vi "mqttClient_ModelController.vi"() -> ()   [LabVIEW 2019]
uses:
  DUT/state -- cluster.ctl
  <vilib>/LabVIEW Open Source Project/OpenSerializer JKI JSON/Serializer.JSON.lvclass
  C:/Program Files (x86)/National Instruments/LabVIEW 2019/vi.lib/LabVIEW Open Source Project/OpenSerializer/Serializer/Serializer.lvclass
  DUT/target -- cluster.ctl
  <vilib>/LabVIEW Open Source Project/MQTT Connection/MQTT_Base/Base Class/MQTT_Base.lvclass/MQTT_Base.ctl
  <vilib>/LabVIEW Open Source Project/MQTT Client/Client class/Client.lvclass/Client.ctl
  <vilib>/LabVIEW Open Source Project/MQTT Control Packets/Control Packets/ControlPacket/QualityOfService -- enum.ctl
  <vilib>/LabVIEW Open Source Project/MQTT Control Packets/Control Packets/ControlPacket/ControlPacket.lvclass/ControlPacket.ctl
  <vilib>/LabVIEW Open Source Project/MQTT Control Packets/Control Packets/CONNECT/ConnectFlags -- cluster.ctl
  <vilib>/numeric/Random Number (Range) DBL.vi
  <vilib>/LabVIEW Open Source Project/MQTT TCP Connection/MQTT_TCP/Connection/TCPConnection.lvclass
  C:/Program Files (x86)/National Instruments/LabVIEW 2019/vi.lib/LabVIEW Open Source Project/MQTT Connection/MQTT_Connection/Connection/Connection.lvclass
  <vilib>/LabVIEW Open Source Project/MQTT Client/Client class/Client.lvclass
  C:/Program Files (x86)/National Instruments/LabVIEW 2019/vi.lib/LabVIEW Open Source Project/MQTT Connection/MQTT_Base/Base Class/MQTT_Base.lvclass
  <vilib>/LabVIEW Open Source Project/OpenSerializer/Serializer.FlattenedString/Serializer.FlattenedString.lvclass
  <vilib>/LabVIEW Open Source Project/MQTT Control Packets/Control Packets/PUBLISH/PUBLISH.lvclass
  C:/Program Files (x86)/National Instruments/LabVIEW 2019/vi.lib/LabVIEW Open Source Project/MQTT Control Packets/Control Packets/ControlPacket/ControlPacket.lvclass
  <vilib>/LabVIEW Open Source Project/OpenSerializer/Serializer/Serializer.lvclass
  <vilib>/LabVIEW Open Source Project/MQTT Connection/MQTT_Base/Base Class/MQTT_Base.lvclass
  <vilib>/LabVIEW Open Source Project/MQTT Control Packets/Control Packets/ControlPacket/ControlPacket.lvclass
  <vilib>/LabVIEW Open Source Project/MQTT Control Packets/Control Packets/CONNECT/CONNECT.lvclass
panel:
  in  "Connection":bool
  out "Last Error":errorcluster
  out "Incoming Payload":string
  out "state":T1 {"measured" format="%.1g"; "setpoint" format="%.1g"}
  # "Native LabVIEW MQTT Client (Model - Controller)"
  # "G Open Source Project for LabVIEW\nhttps://github.com/LabVIEW-Open-Source/MQTT-Client"
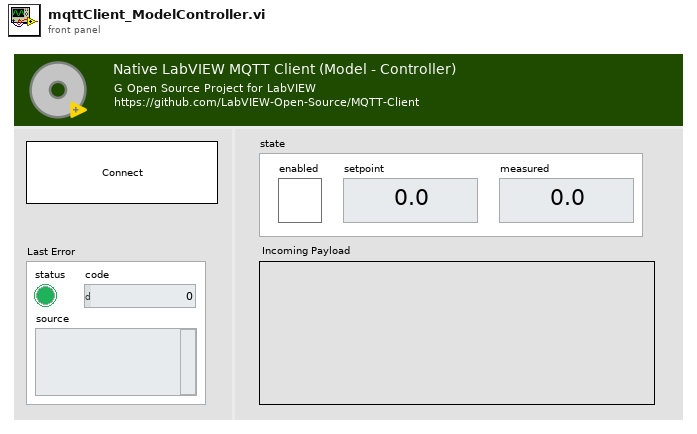
[diagram p1: front panel]
types:
  T1 = typedef "state -- cluster.ctl" = cluster{"enabled":bool, "setpoint":dbl, "measured":dbl}
  T2 = typedef "target -- cluster.ctl" = cluster{"enabled":bool, "setpoint":dbl}
  T3 = cluster{"appName":string, "state":T1, "target":T2}
  T4 = typedef "MQTT Client.lvlib/Client.lvclass/Public Events -- cluster.ctl" = cluster{"Connection Status":refnum<user-event>, "Connected":refnum<user-event>, "Application Message":refnum<user-event>}
  T5 = typedef "MQTT Base.lvlib/MQTT_Base.lvclass/Public Events -- cluster.ctl" = cluster{"Stop Event":refnum<user-event>, "Error Event":refnum<user-event>, "Inbound Message":refnum<user-event>}
  T6 = typedef "MQTT_Control_Packets.lvlib/ControlPacket.lvclass/QualityOfService -- enum.ctl" = enum16{"0 (At Most Once)", "1 (At Least Once)", "2 (Exactly Once)"}
  T7 = typedef "MQTT_Control_Packets.lvlib/CONNECT.lvclass/ConnectFlags -- cluster.ctl" = cluster{"Reserved":bool, "Clean Session":bool, "Will Flag":bool, "Will QoS 1":bool, "Will QoS 2":bool, "Will Retain":bool, "Password Flag":bool, "User Name Flag":bool}
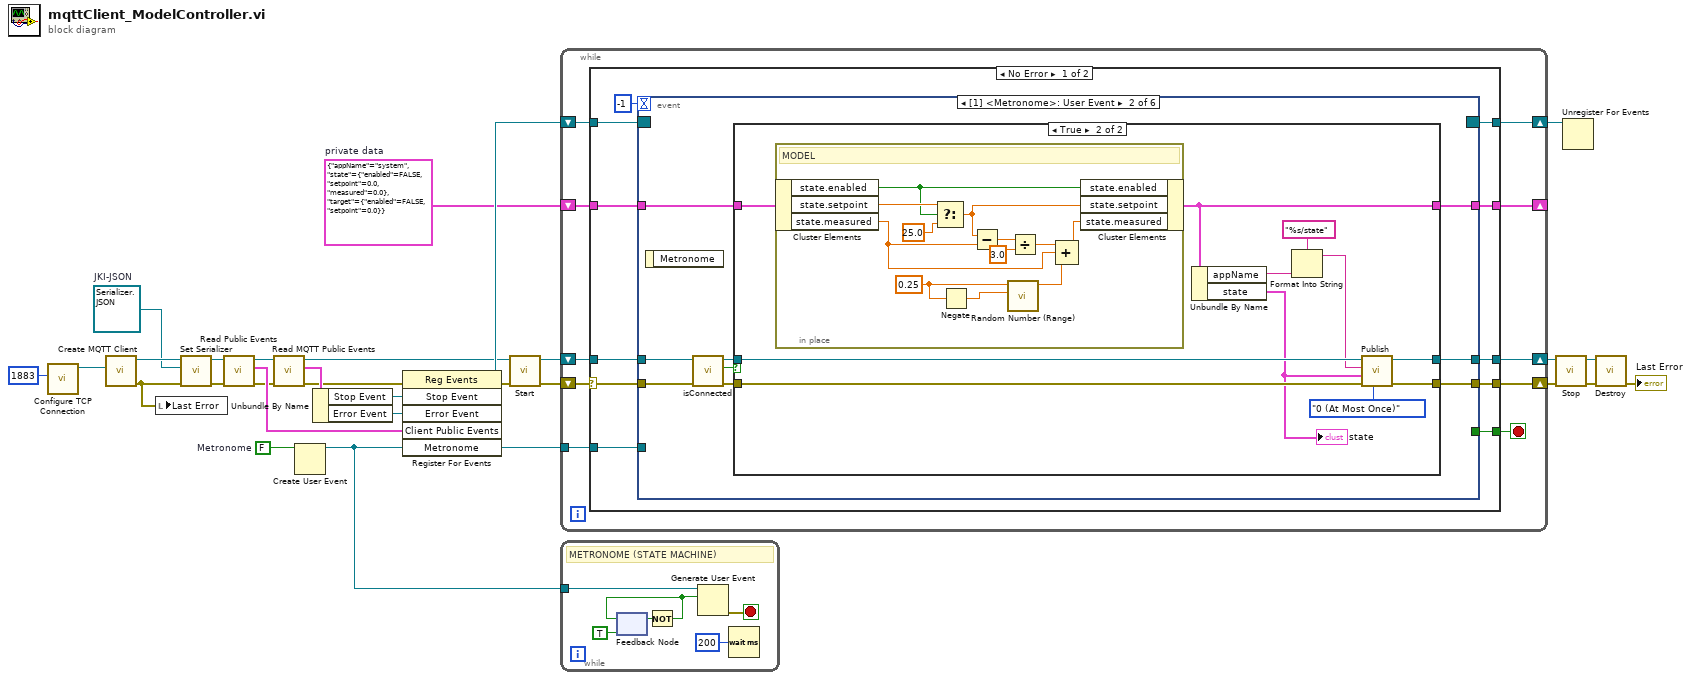
[diagram p0: block diagram]
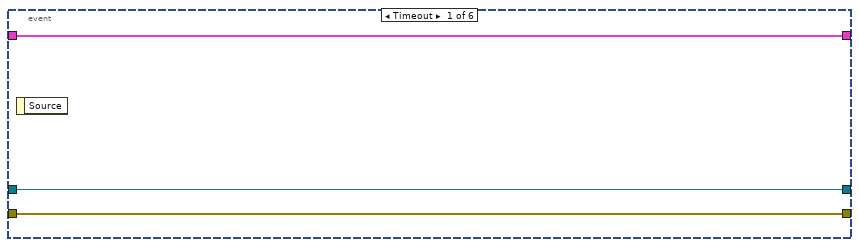
[diagram p2: hidden frame]
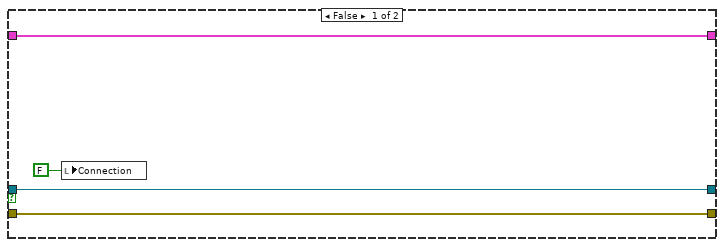
[diagram p3: hidden frame]
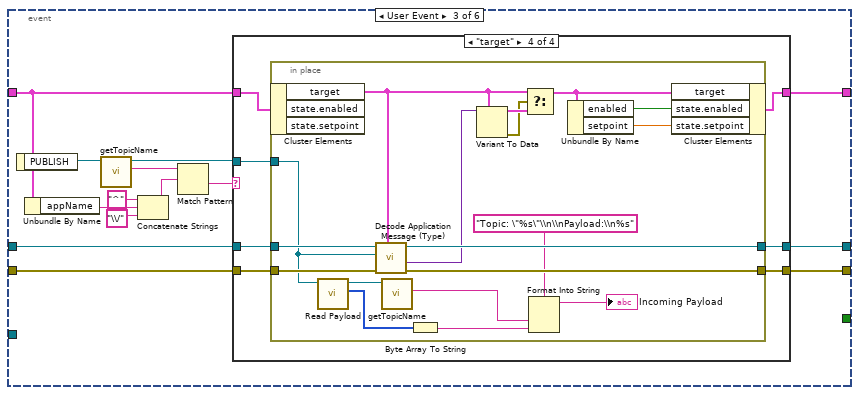
[diagram p4: hidden frame]
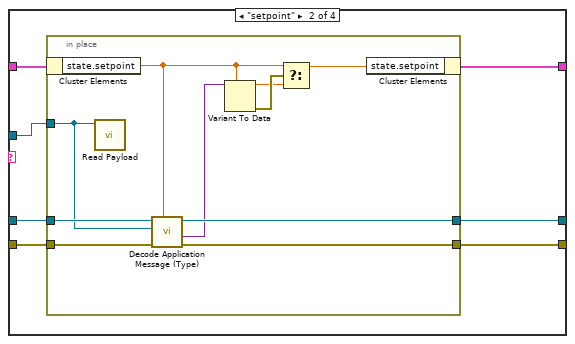
[diagram p6: hidden frame]
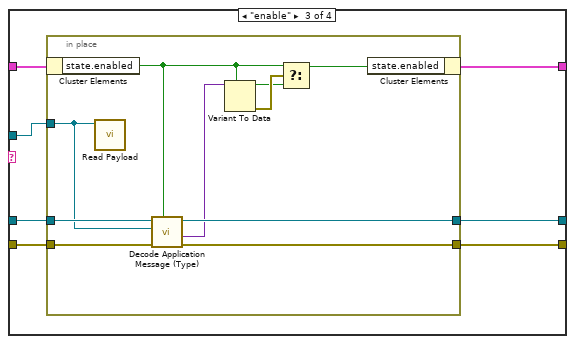
[diagram p7: hidden frame]
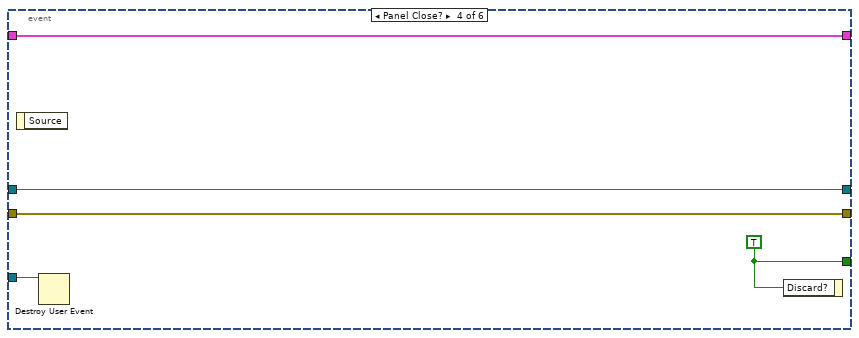
[diagram p8: hidden frame]
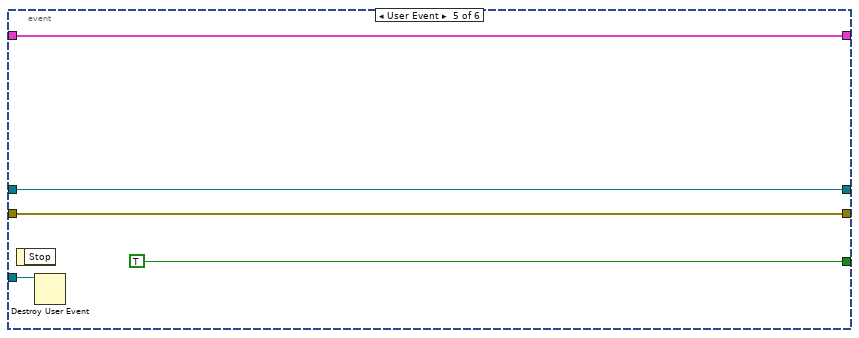
[diagram p9: hidden frame]
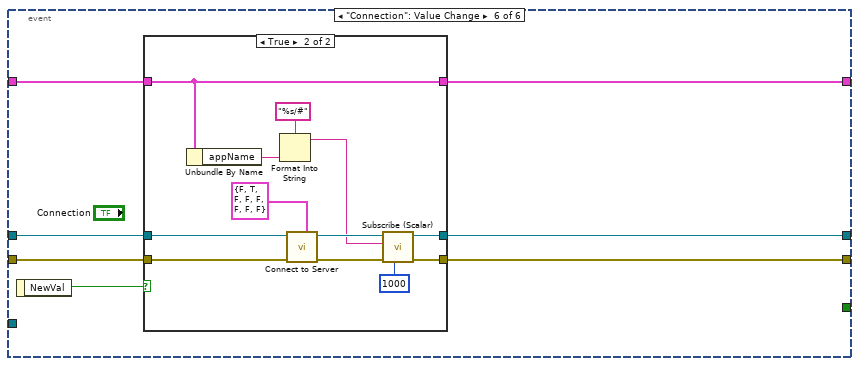
[diagram p10: hidden frame]
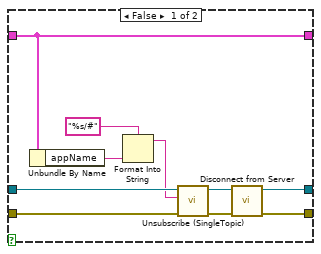
[diagram p11: hidden frame]
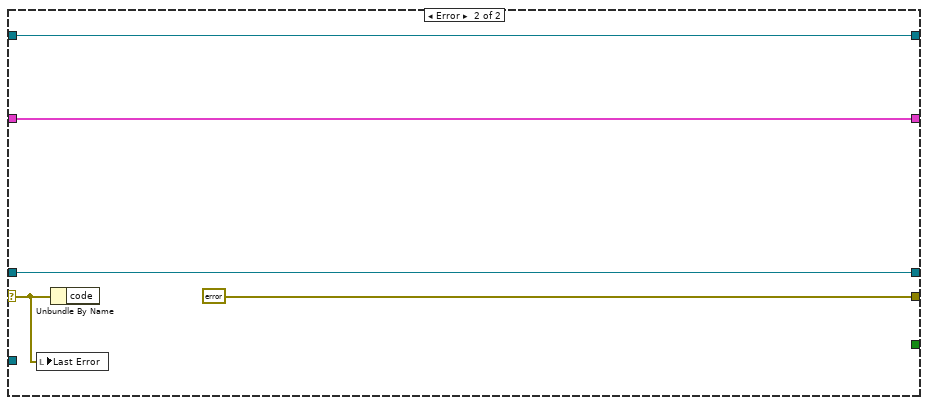
[diagram p12: hidden frame]
diagram:
  w2 = FALSE  # Metronome
  w4 = T3 {"appName"="system", "state"={"enabled"=FALSE, "setpoint"=0.0, "measured"=0.0}, "target"={"enabled"=FALSE, "setpoint"=0.0}}  # private data
  w7 = refnum<class "Serializer.JSON.lvclass"> refnum  # JKI-JSON
  n1 = call <vilib>:"Configure TCP Connection.vi"("remote port (80)"=u16 1883) -> ("TCPConnection"=w11:refnum<class "TCPConnection.lvclass">)  [unwired: 9 in, 1 out]
  n2 = call <vilib>:"Create MQTT Client.vi"("Connection Configuration"=w11) -> ("error out"=w3:errorcluster, "Client out"=w10:refnum<class "Client.lvclass">)  [unwired: 9 in]
  n3 = local write "Last Error"(w3) -> ()
  n4 = call <vilib>:"Set Serializer.vi"("error in (no error)"=w3, "Serializer (default: Flattened String)"=w7, "MQTT_Base"=w10) -> ("error out"=w8:errorcluster, "MQTT_Base out"=w9:refnum<class "Client.lvclass">)  [unwired: 7 in]
  n5 = call <vilib>:"Read Public Events.vi"("error in (no error)"=w8, "Client in"=w9) -> ("error out"=w13:errorcluster, "Client Public Events"=w15:T4, "Client out"=w12:refnum<class "Client.lvclass">)  [unwired: 7 in]
  n6 = call <vilib>:"Read MQTT Public Events.vi"("error in (no error)"=w13, "MQTT_Base in"=w12) -> ("error out"=w14:errorcluster, "MQTT Public Events"=w22:T5, "MQTT_Base out"=w17:refnum<class "Client.lvclass">)  [unwired: 7 in]
  n7 = Create User Event(user event datatype=w2) -> (user event=w1:refnum<user-event>)  [unwired: 1 in, 1 out]
  n8 = Unbundle By Name(w22) -> ("Stop Event"=w20:refnum<user-event>, "Error Event"=w21:refnum<user-event>)
  n9 = register-events(error in=w14, w20, w21, w15, w1) -> (reference out=w18:refnum<event-registration>, error out=w16:errorcluster)  [unwired: 1 in]
  n10 = call <vilib>:"Start.vi"("error in (no error)"=w16, "MQTT_Base in"=w17) -> ("error out"=w5:errorcluster, "MQTT_Base out"=w6:refnum<class "Client.lvclass">)  [unwired: 7 in, 1 out]
  n11 = while {
    shift-right: [w37] -> w19
    shift-left: w18 -> [w38]
    shift-right: [w34] -> w24
    shift-left: w6 -> [w35]
    shift-right: [w36] -> w26
    shift-left: w5 -> [w32]
    shift-right: [w30] -> _
    shift-left: w4 -> [w31]
    tunnel: w1 -> [w29]
    stop <- w33 stop-if-true
    n12 = case shown="No Error" w32 {
      selector: w32 -> [w42 w207]
      tunnel: w38 -> [w49 w206]
      tunnel: [w48 w206] -> w37
      tunnel: [w47 errorcluster {"status"=FALSE, "code"=0, "source"=""} ("error out")] -> w36
      tunnel: w35 -> [w45 w208]
      tunnel: [w44 w208] -> w34
      tunnel: [w43 _] -> w33
      tunnel: w31 -> [w41 w205]
      tunnel: [w40 w205] -> w30
      tunnel: w29 -> [w39 _]
      frame No Error {
        n13 = event shown="[1] <Metronome>: User Event" {
          selector: w49 -> [_ _ _ _ _ _]
          dyn-events: [_ _ _ _ _ _] -> w48
          timeout: -1 -> [_ _ _ _ _ _]
          tunnel: w42 -> [w50 w57 w99 w167 w174 w177]
          tunnel: [w50 w60 w97 w167 w174 w178] -> w47
          tunnel: [_ _ _ w169 TRUE _] -> w43
          tunnel: w45 -> [w51 w59 w100 w168 w172 w181]
          tunnel: [w51 w61 w98 w168 w172 w179] -> w44
          tunnel: w41 -> [w52 w54 w95 w166 w171 w175]
          tunnel: [w52 w53 w96 w166 w171 w176] -> w40
          tunnel: w39 -> [_ _ _ w165 w170 _]
          event Timeout {
            n14 = event-data() -> ()  [unwired: 1 in, 1 out]
          }
          event User Event {
            n15 = event-data() -> ()  [unwired: 1 in, 1 out]
            n16 = call <vilib>:"isConnected.vi"("error in (no error)"=w57, "Client in"=w59) -> ("error out"=w56:errorcluster, "connected"=w55:bool, "Client out"=w58:refnum<class "Client.lvclass">)  [unwired: 7 in]
            n17 = case shown="True" w55 {
              tunnel: [w65 w75] -> w61
              tunnel: [w64 w73] -> w60
              tunnel: w58 -> [w65 w76]
              tunnel: w56 -> [w64 w74]
              tunnel: w54 -> [w62 w69]
              tunnel: [w62 w68] -> w53
              frame False {
                n18 = local write "Connection"(FALSE ("Connection")) -> ()
              }
              frame True {
                n19 = in-place {
                  w78 = 0.25 ("lower bound (0)")
                  # "MODEL"
                  n20 = in-place-cluster #1(w69) -> ("state.enabled"=w86:bool, "state.setpoint"=w87:dbl, "state.measured"=w81:dbl)
                  n21 = Select(t=w87, s=w86, f=25.0) -> (s? t:f=w85:dbl)
                  n22 = Negate(x=w78) -> (-x=w79:dbl)
                  n23 = Subtract(x=w85, y=w81) -> (x-y=w83:dbl)
                  n24 = call-poly <vilib>:"Random Number (Range).vi"("lower bound (0)"=w79, "upper bound (100)"=w78) -> ("number"=w77:dbl)  [unwired: 9 in]
                  n25 = Divide(x=w83, y=3.0 ("f")) -> (x/y=w82:dbl)
                  n26 = Compound Arithmetic op=ADD(w82, w81, w77) -> (w80:dbl)
                  n27 = in-place-cluster #1("state.enabled"=w86, "state.setpoint"=w85, "state.measured"=w80) -> (w68:T3)
                }
                n28 = Unbundle By Name(w68) -> ("appName"=w66:string, "state"=w67:T1)
                "state" <- w67
                n29 = Format Into String(format string="%s/state" ("Topic Name (empty: Payload name)"), w66) -> (resulting string=w70:string)  [unwired: 2 in, 1 out]
                n30 = call <vilib>:"Publish.vi"("QoS"=QualityOfService_--_enum."0 (At Most Once)", "error in (no error)"=w74, "Payload"=w67, "Topic Name (empty: Payload name)"=w70, "Client in"=w76) -> ("error out"=w73:errorcluster, "Client out"=w75:refnum<class "Client.lvclass">)  [unwired: 4 in, 1 out]
              }
            }
          }
          event User Event {
            n31 = event-data() -> ("PUBLISH"=w102:refnum<class "PUBLISH.lvclass">)  [unwired: 1 in]
            n32 = Unbundle By Name(w95) -> ("appName"=w94:string)
            n33 = call <vilib>:"getTopicName.vi"("PUBLISH in"=w102) -> ("Topic"=w90:string, "PUBLISH out"=w101:refnum<class "PUBLISH.lvclass">)  [unwired: 8 in, 1 out]
            n34 = Concatenate Strings("^" ("string"), w94, "\\/" ("string")) -> (w91:string)
            n35 = Match Pattern(string=w90, regular expression=w91) -> (after substring=w89:string)  [unwired: 1 in, 3 out]
            n36 = case shown="\"target\"" w89 {
              tunnel: w101 -> [_ w108 w125 w142]
              tunnel: w100 -> [w105 w110 w127 w144]
              tunnel: w99 -> [w104 w109 w126 w143]
              tunnel: [w105 w107 w124 w141] -> w98
              tunnel: [w104 w106 w123 w140] -> w97
              tunnel: w95 -> [w103 w112 w129 w146]
              tunnel: [w103 w111 w128 w145] -> w96
              frame Default {
              }
              frame "setpoint" {
                n37 = in-place {
                  in-place-border: w110 -> [w122]
                  in-place-border: w109 -> [w121]
                  in-place-border: w108 -> [w113]
                  in-place-border: [w120] -> w107
                  in-place-border: [w119] -> w106
                  n38 = in-place-cluster #2(w112) -> ("state.setpoint"=w115:dbl)
                  n39 = call <vilib>:"Read Payload.vi"("ControlPacket in"=w113) -> ()  [unwired: 9 in, 2 out]
                  n40 = call <vilib>:"Decode Application Message (Type).vi"("Type"=w115, "error in (no error)"=w121, "PUBLISH"=w113, "Client in"=w122) -> ("error out"=w119:errorcluster, "Payload"=w118:variant, "Client out"=w120:refnum<class "Client.lvclass">)  [unwired: 4 in, 1 out]
                  n41 = Variant To Data(type=w115, Variant=w118) -> (data=w116:dbl, error out=w117:errorcluster)  [unwired: 1 in]
                  n42 = Select(t=w115, s=w117, f=w116) -> (s? t:f=w114:dbl)
                  n43 = in-place-cluster #2("state.setpoint"=w114) -> (w111:T3)
                }
              }
              frame "enable" {
                n44 = in-place {
                  in-place-border: w127 -> [w139]
                  in-place-border: w126 -> [w138]
                  in-place-border: w125 -> [w130]
                  in-place-border: [w137] -> w124
                  in-place-border: [w136] -> w123
                  n45 = in-place-cluster #3(w129) -> ("state.enabled"=w132:bool)
                  n46 = call <vilib>:"Read Payload.vi"("ControlPacket in"=w130) -> ()  [unwired: 9 in, 2 out]
                  n47 = call <vilib>:"Decode Application Message (Type).vi"("Type"=w132, "error in (no error)"=w138, "PUBLISH"=w130, "Client in"=w139) -> ("error out"=w136:errorcluster, "Payload"=w135:variant, "Client out"=w137:refnum<class "Client.lvclass">)  [unwired: 4 in, 1 out]
                  n48 = Variant To Data(type=w132, Variant=w135) -> (data=w133:bool, error out=w134:errorcluster)  [unwired: 1 in]
                  n49 = Select(t=w132, s=w134, f=w133) -> (s? t:f=w131:bool)
                  n50 = in-place-cluster #3("state.enabled"=w131) -> (w128:T3)
                }
              }
              frame "target" {
                n51 = in-place {
                  in-place-border: w144 -> [w164]
                  in-place-border: w143 -> [w163]
                  in-place-border: w142 -> [w157]
                  in-place-border: [w162] -> w141
                  in-place-border: [w161] -> w140
                  n52 = in-place-cluster #4(w146) -> ("target"=w158:T2)  [unwired: 2 out]
                  n53 = call <vilib>:"Read Payload.vi"("ControlPacket in"=w157) -> ("Payload"=w156:u8[], "ControlPacket out"=w151:refnum<class "PUBLISH.lvclass">)  [unwired: 9 in]
                  n54 = call <vilib>:"Decode Application Message (Type).vi"("Type"=w158, "error in (no error)"=w163, "PUBLISH"=w157, "Client in"=w164) -> ("error out"=w161:errorcluster, "Payload"=w160:variant, "Client out"=w162:refnum<class "Client.lvclass">)  [unwired: 4 in, 1 out]
                  n55 = call <vilib>:"getTopicName.vi"("PUBLISH in"=w151) -> ("Topic"=w149:string)  [unwired: 8 in, 2 out]
                  n56 = Byte Array To String(unsigned byte array=w156) -> (string=w148:string)
                  n57 = Variant To Data(type=w158, Variant=w160) -> (data=w159:T2, error out=w152:errorcluster)  [unwired: 1 in]
                  n58 = Select(t=w158, s=w152, f=w159) -> (s? t:f=w155:T2)
                  n59 = Format Into String(format string="Topic: \"%s\"\\n\\nPayload:\\n%s", w149, w148) -> (resulting string=→"Incoming Payload":string)  [unwired: 2 in, 1 out]
                  n60 = Unbundle By Name(w155) -> ("enabled"=w154:bool, "setpoint"=w153:dbl)
                  n61 = in-place-cluster #4("target"=w155, "state.enabled"=w154, "state.setpoint"=w153) -> (w145:T3)
                }
              }
            }
          }
          event Panel Close? {
            w169 = TRUE
            n62 = event-data() -> ()  [unwired: 1 in, 1 out]
            n63 = Destroy User Event(user event=w165) -> ()  [unwired: 1 in, 1 out]
            n64 = event-data("Discard?"=w169) -> ()  [unwired: 1 in, 1 out]
          }
          event User Event {
            n65 = event-data() -> ()  [unwired: 1 in, 1 out]
            n66 = Destroy User Event(user event=w170) -> ()  [unwired: 1 in, 1 out]
          }
          event "Connection": Value Change {
            n67 = event-data() -> ("NewVal"=w180:bool)  [unwired: 1 in]
            n68 = case shown="True" w180 {
              tunnel: w181 -> [w188 w203]
              tunnel: [w191 w196] -> w179
              tunnel: [w190 w198] -> w178
              tunnel: w177 -> [w186 w202]
              tunnel: [w183 w201] -> w176
              tunnel: w175 -> [w183 w201]
              frame False {
                n69 = Unbundle By Name(w183) -> ("appName"=w185:string)
                n70 = Format Into String(format string="%s/#" ("Topic Name (empty: Payload name)"), w185) -> (resulting string=w182:string)  [unwired: 2 in, 1 out]
                n71 = call <vilib>:"Unsubscribe (SingleTopic).vi"("error in (no error)"=w186, "Topic Filter"=w182, "MQTT_Base in"=w188) -> ("error out"=w187:errorcluster, "MQTT_Base out"=w189:refnum<class "Client.lvclass">)  [unwired: 6 in, 1 out]
                n72 = call <vilib>:"Disconnect from Server.vi"("error in (no error)"=w187, "Client in"=w189) -> ("error out"=w190:errorcluster, "Client out"=w191:refnum<class "Client.lvclass">)  [unwired: 7 in, 1 out]
              }
              frame True {
                n73 = Unbundle By Name(w201) -> ("appName"=w194:string)
                n74 = Format Into String(format string="%s/#" ("Topic Name (empty: Payload name)"), w194) -> (resulting string=w192:string)  [unwired: 2 in, 1 out]
                n75 = call <vilib>:"Connect to Server.vi"("Connect Flags"=T7 {"Reserved"=FALSE, "Clean Session"=TRUE, "Will Flag"=FALSE, "Will QoS 1"=FALSE, "Will QoS 2"=FALSE, "Will Retain"=FALSE, "Password Flag"=FALSE, "User Name Flag"=FALSE}, "error in (no error)"=w202, "Client in"=w203) -> ("error out"=w195:errorcluster, "Client out"=w197:refnum<class "Client.lvclass">)  [unwired: 5 in, 2 out]
                n76 = call <vilib>:"Subscribe (Scalar).vi"("timeout (1000ms)"=1000 ("timeout (100ms)"), "error in (no error)"=w195, "Topic Filter"=w192, "Client in"=w197) -> ("error out"=w198:errorcluster, "Client out"=w196:refnum<class "Client.lvclass">)  [unwired: 5 in, 1 out]
              }
            }
          }
        }
      }
      frame Error {
        n77 = local write "Last Error"(w207) -> ()
        n78 = Unbundle By Name(w207) -> ()  [unwired: 1 out]
      }
    }
  }
  n79 = while {
    tunnel: w1 -> [w214]
    stop <- w213 stop-if-true
    # "METRONOME (STATE MACHINE)"
    n80 = feedback #5(TRUE) -> (w211:bool)
    n81 = Not(x=w211) -> (.not. x?=w210:bool)
    n82 = feedback-in #5(w210) -> ()
    n83 = Generate User Event(user event=w214, event data cluster=w210) -> (error out=w213:errorcluster)  [unwired: 2 in, 1 out]
    n84 = Wait (ms)(milliseconds to wait=u32 200) -> ()  [unwired: 1 out]
  }
  n85 = call <vilib>:"Stop.vi"("error in (no error)"=w26, "MQTT_Base in"=w24) -> ("error out"=w25:errorcluster, "MQTT_Base out"=w23:refnum<class "Client.lvclass">)  [unwired: 7 in, 1 out]
  n86 = Unregister For Events(event registration refnum=w19) -> ()  [unwired: 1 in, 1 out]
  n87 = call <vilib>:"Destroy.vi"("error in (no error)"=w25, "MQTT_Base in"=w23) -> ("error out"=→"Last Error":errorcluster)  [unwired: 8 in, 1 out]
